vi "OPCUA to LVData.vi"(8 "Error In":errorcluster, 10 "DataType":u32, 11 "OPCUA Variant in":variant) -> (0 "Error Out":errorcluster, 3 "OPCUA Variant out":variant)   [LabVIEW 2015, in "CS++OPCUAInterface.lvlib" / "CS++OPCUAInterface.lvclass"]
uses:
  CS++OPCUAInterface.lvclass
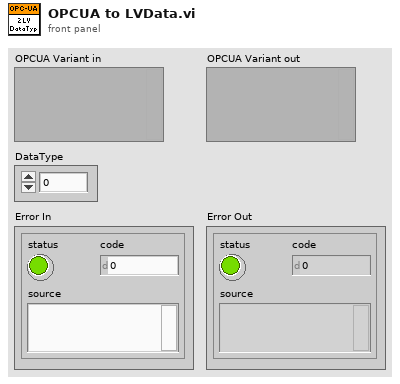
[diagram p1: front panel]
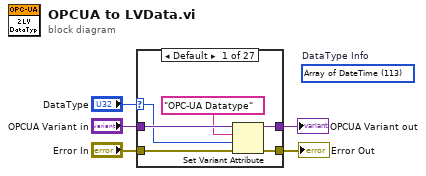
[diagram p0: block diagram]
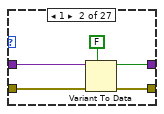
[diagram p2: hidden frame]
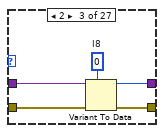
[diagram p3: hidden frame]
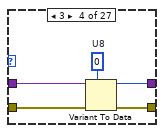
[diagram p4: hidden frame]
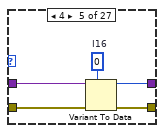
[diagram p5: hidden frame]
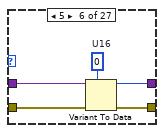
[diagram p6: hidden frame]
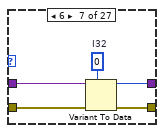
[diagram p7: hidden frame]
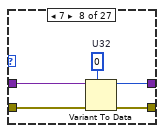
[diagram p8: hidden frame]
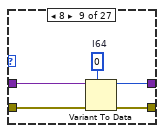
[diagram p9: hidden frame]
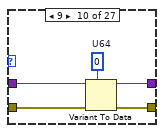
[diagram p10: hidden frame]
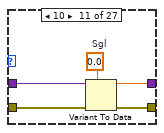
[diagram p11: hidden frame]
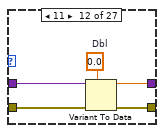
[diagram p12: hidden frame]
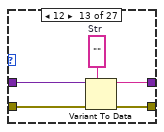
[diagram p13: hidden frame]
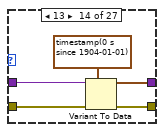
[diagram p14: hidden frame]
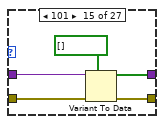
[diagram p15: hidden frame]
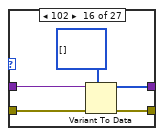
[diagram p16: hidden frame]
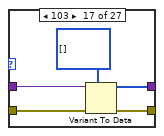
[diagram p17: hidden frame]
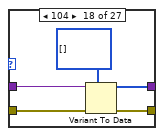
[diagram p18: hidden frame]
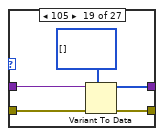
[diagram p19: hidden frame]
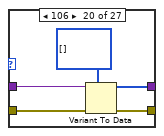
[diagram p20: hidden frame]
diagram:
  (unwired) u32 113 items=["Boolean"=1, "SByte"=2, "Byte"=3, "Int16"=4, "UInt16"=5, "Int32"=6, "UInt32"=7, "Int64"=8, "UInt64"=9, "Float"=10, "Double"=11, "String"=12, "DateTime"=13, "ByteString"=15, "Array of Boolean"=101, "Array of SByte"=102, "Array of Byte"=103, "Array of Int16"=104, "Array of UInt16"=105, "Array of Int32"=106, "Array of UInt32"=107, "Array of Int64"=108, "Array of UInt64"=109, "Array of Float"=110, "Array of Double"=111, "Array of String"=112, "Array of DateTime"=113, "Array of ByteString"=115]  # DataType Info
  n1 = case shown="Default" "DataType" {
    selector: "DataType" -> [w6 _ _ _ _ _ _ _ _ _ _ _ _ _ _ _ _ _ _ _ _ _ _ _ _ _ _]
    tunnel: "OPCUA Variant in" -> [w9 w16 w21 w26 w31 w36 w41 w46 w51 w56 w61 w66 w71 w76 w81 w86 w91 w96 w101 w106 w111 w116 w121 w126 w131 w136 w141]
    tunnel: "Error In" -> [w11 w15 w20 w25 w30 w35 w40 w45 w50 w55 w60 w65 w70 w75 w80 w85 w90 w95 w100 w105 w110 w115 w120 w125 w130 w135 w140]
    tunnel: [w10 w14 w19 w24 w29 w34 w39 w44 w49 w54 w59 w64 w69 w74 w79 w84 w89 w94 w99 w104 w109 w114 w119 w124 w129 w134 w139] -> w3
    tunnel: [w8 w13 w18 w23 w28 w33 w38 w43 w48 w53 w58 w63 w68 w73 w78 w83 w88 w93 w98 w103 w108 w113 w118 w123 w128 w133 w138] -> w2
    frame Default {
      n2 = Set Variant Attribute(Variant=w9, name="OPC-UA Datatype", value=w6, error in=w11) -> (Variant out=w8:variant, error out=w10:errorcluster)  [unwired: 1 out]
    }
    frame 1 {
      n3 = Variant To Data(error in=w15, type=FALSE, Variant=w16) -> (data=w13:bool, error out=w14:errorcluster)
    }
    frame 2 {
      w17 = i8 0  # I8
      n4 = Variant To Data(error in=w20, type=w17, Variant=w21) -> (data=w18:i8, error out=w19:errorcluster)
    }
    frame 3 {
      w22 = u8 0  # U8
      n5 = Variant To Data(error in=w25, type=w22, Variant=w26) -> (data=w23:u8, error out=w24:errorcluster)
    }
    frame 4 {
      w27 = i16 0  # I16
      n6 = Variant To Data(error in=w30, type=w27, Variant=w31) -> (data=w28:i16, error out=w29:errorcluster)
    }
    frame 5 {
      w32 = u16 0  # U16
      n7 = Variant To Data(error in=w35, type=w32, Variant=w36) -> (data=w33:u16, error out=w34:errorcluster)
    }
    frame 6 {
      w37 = 0  # I32
      n8 = Variant To Data(error in=w40, type=w37, Variant=w41) -> (data=w38:i32, error out=w39:errorcluster)
    }
    frame 7 {
      w42 = u32 0  # U32
      n9 = Variant To Data(error in=w45, type=w42, Variant=w46) -> (data=w43:u32, error out=w44:errorcluster)
    }
    frame 8 {
      w47 = i64 0  # I64
      n10 = Variant To Data(error in=w50, type=w47, Variant=w51) -> (data=w48:i64, error out=w49:errorcluster)
    }
    frame 9 {
      w52 = u64 0  # U64
      n11 = Variant To Data(error in=w55, type=w52, Variant=w56) -> (data=w53:u64, error out=w54:errorcluster)
    }
    frame 10 {
      w57 = sgl 0.0  # Sgl
      n12 = Variant To Data(error in=w60, type=w57, Variant=w61) -> (data=w58:sgl, error out=w59:errorcluster)
    }
    frame 11 {
      w62 = 0.0  # Dbl
      n13 = Variant To Data(error in=w65, type=w62, Variant=w66) -> (data=w63:dbl, error out=w64:errorcluster)
    }
    frame 12 {
      w67 = ""  # Str
      n14 = Variant To Data(error in=w70, type=w67, Variant=w71) -> (data=w68:string, error out=w69:errorcluster)
    }
    frame 13 {
      n15 = Variant To Data(error in=w75, type=timestamp(0 s since 1904-01-01) ("time stamp"), Variant=w76) -> (data=w73:timestamp, error out=w74:errorcluster)
    }
    frame 101 {
      n16 = Variant To Data(error in=w80, type=bool[] [], Variant=w81) -> (data=w78:bool[], error out=w79:errorcluster)
    }
    frame 102 {
      n17 = Variant To Data(error in=w85, type=i8[] [], Variant=w86) -> (data=w83:i8[], error out=w84:errorcluster)
    }
    frame 103 {
      n18 = Variant To Data(error in=w90, type=u8[] [], Variant=w91) -> (data=w88:u8[], error out=w89:errorcluster)
    }
    frame 104 {
      n19 = Variant To Data(error in=w95, type=i16[] [], Variant=w96) -> (data=w93:i16[], error out=w94:errorcluster)
    }
    frame 105 {
      n20 = Variant To Data(error in=w100, type=u16[] [], Variant=w101) -> (data=w98:u16[], error out=w99:errorcluster)
    }
    frame 106 {
      n21 = Variant To Data(error in=w105, type=i32[] [], Variant=w106) -> (data=w103:i32[], error out=w104:errorcluster)
    }
    frame 107 {
      n22 = Variant To Data(error in=w110, type=u32[] [], Variant=w111) -> (data=w108:u32[], error out=w109:errorcluster)
    }
    frame 108 {
      n23 = Variant To Data(error in=w115, type=i64[] [], Variant=w116) -> (data=w113:i64[], error out=w114:errorcluster)
    }
    frame 109 {
      n24 = Variant To Data(error in=w120, type=u64[] [], Variant=w121) -> (data=w118:u64[], error out=w119:errorcluster)
    }
    frame 110 {
      n25 = Variant To Data(error in=w125, type=sgl[] [], Variant=w126) -> (data=w123:sgl[], error out=w124:errorcluster)
    }
    frame 111 {
      n26 = Variant To Data(error in=w130, type=dbl[] [], Variant=w131) -> (data=w128:dbl[], error out=w129:errorcluster)
    }
    frame 112 {
      n27 = Variant To Data(error in=w135, type=string[] [], Variant=w136) -> (data=w133:string[], error out=w134:errorcluster)
    }
    frame 113 {
      n28 = Variant To Data(error in=w140, type=timestamp[] [], Variant=w141) -> (data=w138:timestamp[], error out=w139:errorcluster)
    }
  }
  "OPCUA Variant out" <- w2
  "Error Out" <- w3
